vi "replaceScriptEvent.vi"(6 "delay events":bool, 8 "error in (no error)":errorcluster, 9 "index":i32, 10 "ScriptEvent":refnum<class "ScriptEvent.lvclass">, 11 "ScriptEventList in":refnum<class "ScriptEventList.lvclass">) -> (0 "error out":errorcluster, 3 "ScriptEventList out":refnum<class "ScriptEventList.lvclass">)   [LabVIEW 2011, in "Tools.lvlib" / "Scripting.lvlib" / "ScriptEventList.lvclass"]
uses:
  ScriptEventList.lvclass
  ScriptEvent.lvclass
  ScriptEventList.lvclass/ScriptEventList.ctl
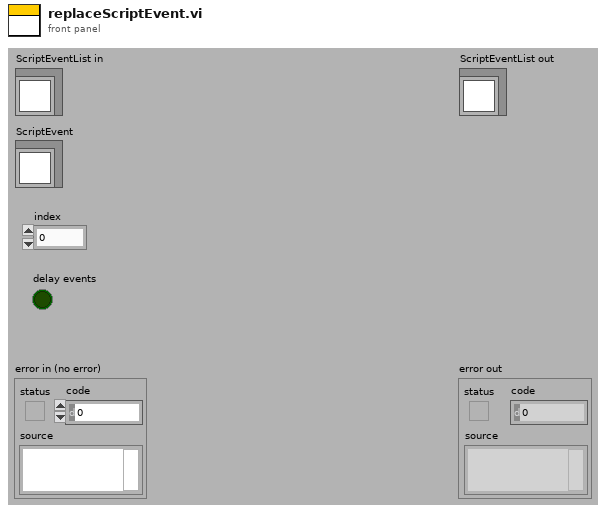
[diagram p1: front panel]
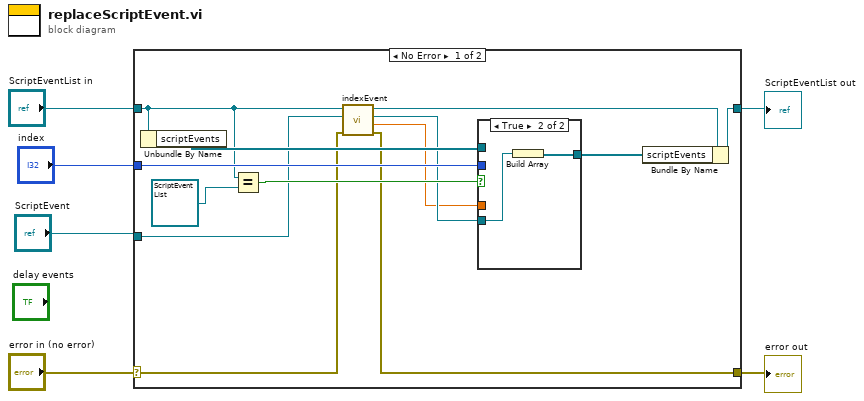
[diagram p0: block diagram]
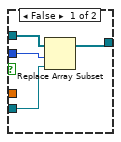
[diagram p2: hidden frame]
diagram:
  n1 = case shown="No Error" "error in (no error)" {
    selector: "error in (no error)" -> [w9 w27]
    tunnel: [w8 w27] -> w5
    tunnel: [w10 w26] -> w3
    tunnel: "ScriptEventList in" -> [w14 w26]
    tunnel: "index" -> [w18 _]
    tunnel: "ScriptEvent" -> [w13 _]
    frame No Error {
      n2 = Unbundle By Name(w14) -> ("scriptEvents"=w19:refnum<class "ScriptEvent.lvclass">[])
      n3 = Equal?(x=w14, y=refnum<class "ScriptEventList.lvclass"> refnum ("Tools.lvlib:Scripting.lvlib:ScriptEventList.lvclass")) -> (x = y?=w16:bool)
      n4 = call "indexEvent.vi"("error in (no error)"=w9, "ScriptEvent"=w13, "ScriptEventList in"=w14) -> ("error out"=w8:errorcluster, "eventId"=w7:dbl, "ScriptEvent out"=w12:refnum<class "ScriptEvent.lvclass">, "ScriptEventList out"=w11:refnum<class "ScriptEventList.lvclass">)  [unwired: 5 in]
      n5 = case shown="True" w16 {
        tunnel: w19 -> [w23 _]
        tunnel: w18 -> [w22 _]
        tunnel: w12 -> [w21 w24]
        tunnel: [w20 w25] -> w17
        tunnel: w7 -> [_ _]
        frame False {
          n6 = Replace Array Subset(array=w23, new element=w21, index=w22) -> (w20:refnum<class "ScriptEvent.lvclass">[])
        }
        frame True {
          n7 = Build Array(w24) -> (w25:refnum<class "ScriptEvent.lvclass">[])
        }
      }
      n8 = Bundle By Name(cluster=w11, "scriptEvents"=w17) -> (w10:refnum<class "ScriptEventList.lvclass">)
    }
    frame Error {
    }
  }
  "error out" <- w5
  "ScriptEventList out" <- w3
